vi "CommandResponse.Create.vi"(8 "error in (no error)":errorcluster, 10 "Signals":T1 {"Response"."Byte Order" items=["Little Endian", "Big Endian"]; "Response"."Data Type" items=["Signed", "Unsigned", "IEEE Float"]; "Cmd"."Byte Order" items=["Little Endian", "Big Endian"]; "Cmd"."Data Type" items=["Signed", "Unsigned", "IEEE Float"]}, 11 "New NodeID":u64) -> (0 "error out":errorcluster)   [LabVIEW 2019, in "Diagnostics Addon System Explorer.lvlib"]
uses:
  Diagnostics Addon System Explorer.lvlib
  Types/CmdResp.Export.ctl
  Shared/Types/Signal.ctl
  Shared/SubVIs/Constants.vi
  Shared/Diagnostics Addon Shared.lvlib
  <vilib>/NI/NI VeriStand Advanced SysDef API/SysDef API/Advanced System Definition.lvlib
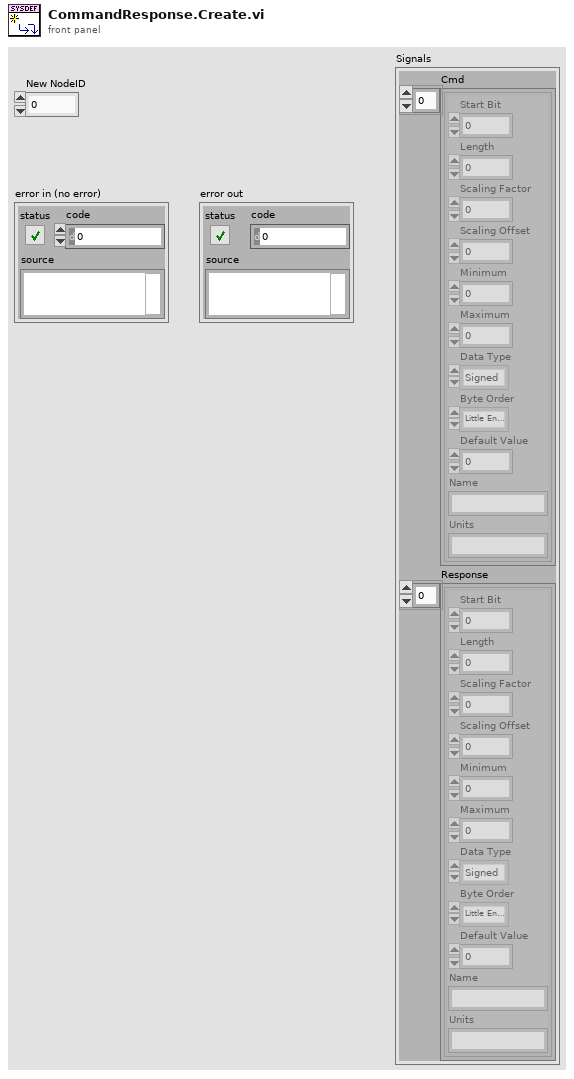
[diagram p1: front panel]
types:
  T1 = typedef "Diagnostics Addon System Explorer.lvlib/CmdResp.Export.ctl" = cluster{"Cmd":T2[], "Response":T2[]}
  T2 = typedef "Diagnostics Addon Shared.lvlib/Signal.ctl" = cluster{"Start Bit":u32, "Length":u32, "Scaling Factor":dbl, "Scaling Offset":dbl, "Minimum":dbl, "Maximum":dbl, "Data Type":u32, "Byte Order":u32, "Default Value":dbl, "Name":string, "Units":string}
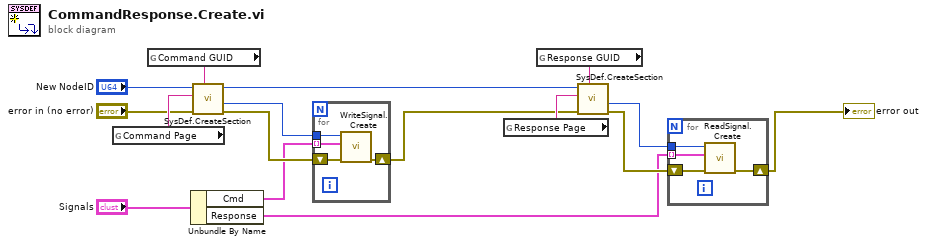
[diagram p0: block diagram]
diagram:
  n1 = global read "Constants.vi" "Command Page"() -> (w13:string)
  n2 = global read "Constants.vi" "Command GUID"() -> (w14:string)
  n3 = Unbundle By Name("Signals") -> ("Cmd"=w2:T2[], "Response"=w1:T2[])
  n4 = call <vilib>:"SysDef.CreateSection.vi"("GUID"=w14, "error in (no error)"="error in (no error)", "Name"=w13, "nodeID"="New NodeID") -> ("error out"=w5:errorcluster, "New NodeID"=w9:u64, "nodeID out"=w10:u64)  [unwired: 4 in, 1 out]
  n5 = for {
    tunnel: w9 -> [w20]
    shift-right: [w18] -> w4
    shift-left: w5 -> [w19]
    tunnel: w2 -> [w17] mode=indexing
    n6 = call "WriteSignal.Create.vi"("error in (no error)"=w19, "Signal Parameters"=w17, "Section Ptr"=w20) -> ("error out"=w18:errorcluster)  [unwired: 7 in, 1 out]
  }
  n7 = global read "Constants.vi" "Response Page"() -> (w16:string)
  n8 = global read "Constants.vi" "Response GUID"() -> (w15:string)
  n9 = call <vilib>:"SysDef.CreateSection.vi"("GUID"=w15, "error in (no error)"=w4, "Name"=w16, "nodeID"=w10) -> ("error out"=w7:errorcluster, "New NodeID"=w8:u64)  [unwired: 4 in, 2 out]
  n10 = for {
    tunnel: w8 -> [w24]
    shift-right: [w22] -> w6
    shift-left: w7 -> [w23]
    tunnel: w1 -> [w21] mode=indexing
    n11 = call "ReadSignal.Create.vi"("error in (no error)"=w23, "Signal Parameters"=w21, "Section Ptr"=w24) -> ("error out"=w22:errorcluster)  [unwired: 7 in, 1 out]
  }
  "error out" <- w6
